vi "Cálculo da nota de vf.vi"() -> ()   [LabVIEW 2018]
panel:
  out "Média VE":dbl format="%#_13g"
  in  "VETOR VE":dbl[](array[numeric])
  in  "VC":dbl format="%#_13g"
  out "VF":dbl format="%#_13g"
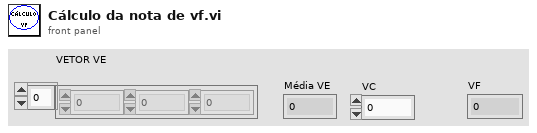
[diagram p1: front panel]
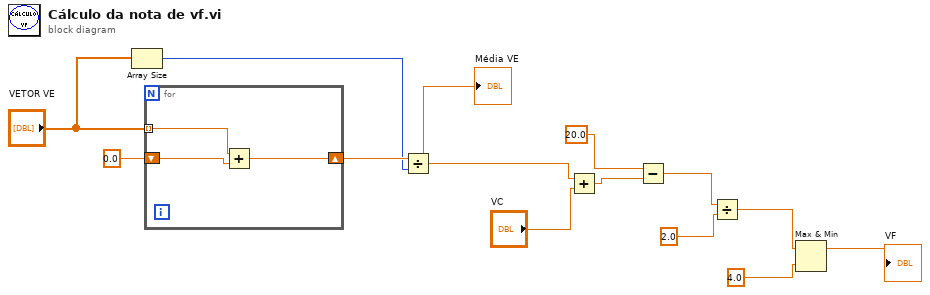
[diagram p0: block diagram]
diagram:
  n1 = Array Size(array="VETOR VE") -> (size(s)=w3:i32)
  n2 = for {
    tunnel: "VETOR VE" -> [w16] mode=indexing
    shift-right: [w14] -> w5
    shift-left: 0.0 -> [w15]
    n3 = Add(x=w16, y=w15) -> (x+y=w14:dbl)
  }
  n4 = Divide(x=w5, y=w3) -> (x/y=w1:dbl)
  "Média VE" <- w1
  n5 = Add(x=w1, y="VC") -> (x+y=w8:dbl)
  n6 = Subtract(x=20.0, y=w8) -> (x-y=w10:dbl)
  n7 = Divide(x=w10, y=2.0) -> (x/y=w12:dbl)
  n8 = Max & Min(x=w12, y=4.0) -> (max(x,y)=→"VF":dbl)  [unwired: 1 out]
